vi "Distance Calcv2.vi"(1 "Particle Points":dbl[][](array[numeric])) -> (0 "Output Distance Array":dbl[](array[numeric]))   [LabVIEW 2014]
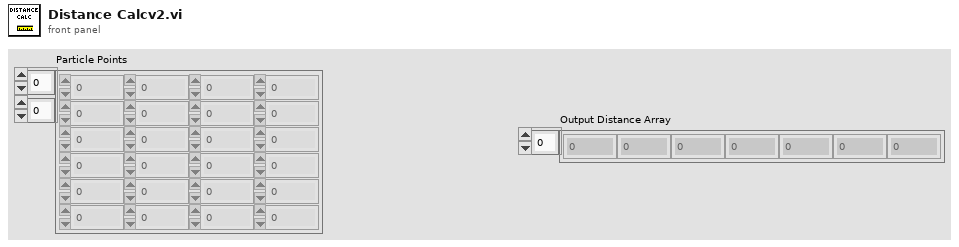
[diagram p1: front panel]
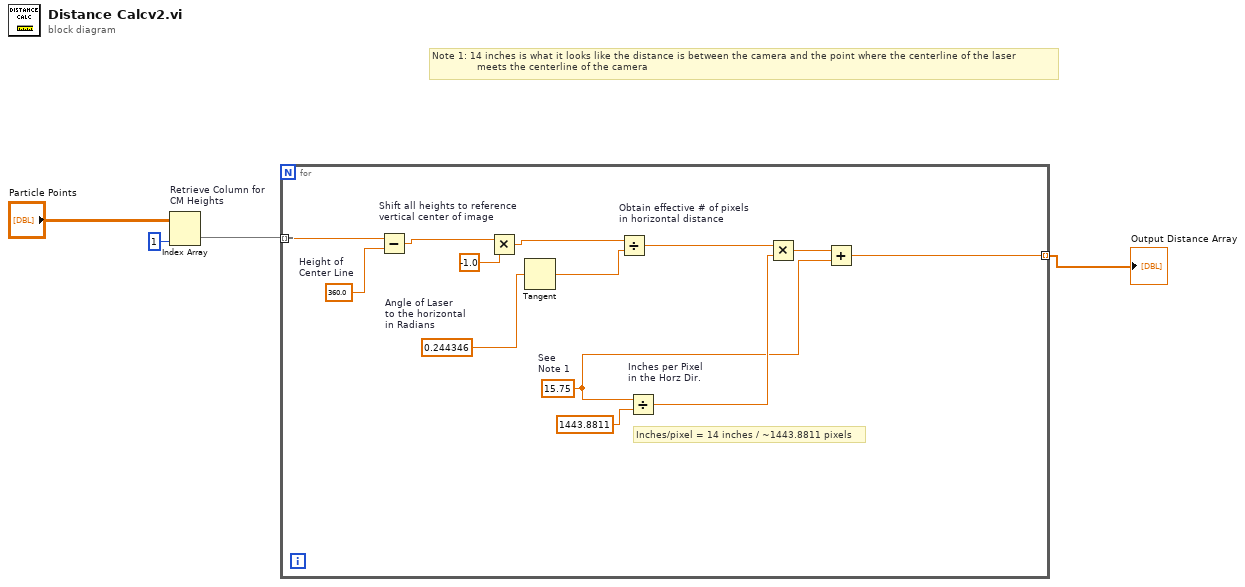
[diagram p0: block diagram]
diagram:
  # "Note 1: 14 inches is what it looks like the distance is between the camera and the point where the centerline of the laser\n               meets the centerline of the camera"
  n1 = Index Array "Retrieve Column for \nCM Heights"(array="Particle Points", index (col)=1 ("disabled index (col)")) -> (element=w2:dbl[])  [unwired: 1 in]
  n2 = for {
    tunnel: w2 -> [w17] mode=indexing
    tunnel: [w11] -> w1 mode=indexing
    w8 = 15.75  # See  Note 1
    w15 = 0.244346  # Angle of Laser to the horizontal in Radians
    w16 = 360.0  # Height of  Center Line
    # "Inches/pixel = 14 inches / ~1443.8811 pixels"
    n3 = Subtract "Shift all heights to reference\nvertical center of image"(x=w17, y=w16) -> (x-y=w7:dbl)
    n4 = Multiply(x=w7, y=-1.0) -> (x*y=w5:dbl)
    n5 = Tangent(1:w15) -> (0:w14:dbl)
    n6 = Divide "Obtain effective # of pixels\nin horizontal distance"(x=w5, y=w14) -> (x/y=w13:dbl)
    n7 = Divide "Inches per Pixel\nin the Horz Dir."(x=w8, y=1443.8811) -> (x/y=w9:dbl)
    n8 = Multiply(x=w13, y=w9) -> (x*y=w12:dbl)
    n9 = Add(x=w12, y=w8) -> (x+y=w11:dbl)
  }
  "Output Distance Array" <- w1
